vi "ULx Write (Analog 1D DBL 1Chan NSamp).vi"(0 "task in":refnum<k24>, 1 "auto start":bool, 7 "data":dbl[](array[numeric]) format="%0.2f", 9 "timeout":dbl=10.0 format="%_4g", 11 "error in":errorcluster) -> (4 "task out":refnum<k24>, 10 "number of samples written per channel":u32, 15 "error out":errorcluster)   [LabVIEW 2020]
doc: "Writes one or more floating-point samples to a task that contains a single analog output channel."
uses:
  C:/Users/William/Documents/LV 2020 builds/LeaktestDAQ/Source-v33/ULx_LV.dll
  ULx_LV.dll
panel:
  # "sample #"
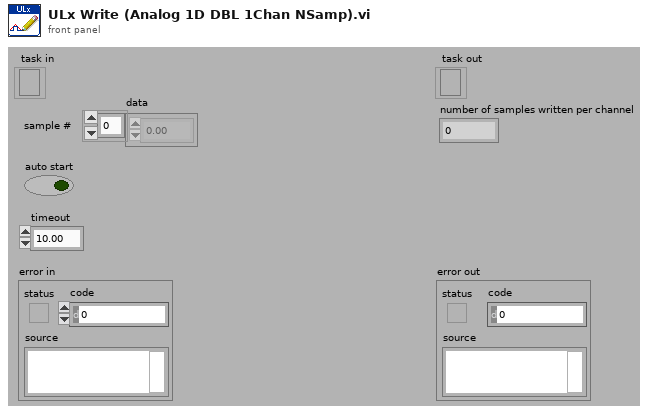
[diagram p1: front panel]
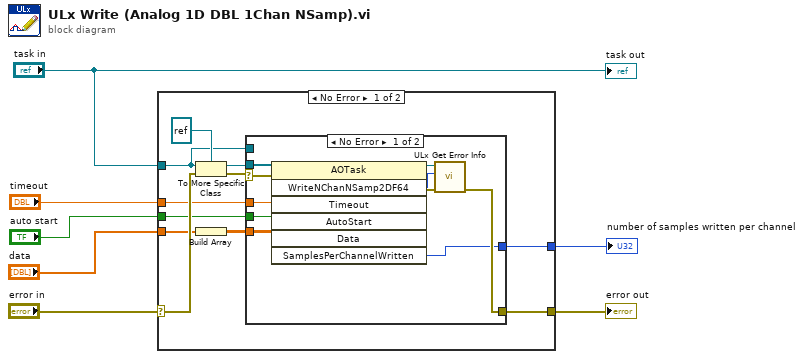
[diagram p0: block diagram]
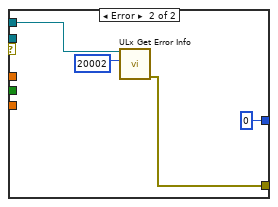
[diagram p2: hidden frame]
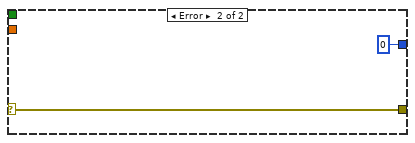
[diagram p3: hidden frame]
diagram:
  n1 = case shown="No Error" "error in" {
    selector: "error in" -> [w18 w34]
    tunnel: "task in" -> [w12 _]
    tunnel: "timeout" -> [w14 _]
    tunnel: [w13 w34] -> w5
    tunnel: "data" -> [w8 _]
    tunnel: "auto start" -> [w11 _]
    tunnel: [w10 0 ("SamplesPerChannelWritten")] -> w1
    frame No Error {
      n2 = To More Specific Class(target class=refnum<k24> refnum, reference=w12, error in=w18) -> (specific class reference=w15:refnum<k24>, error out=w16:errorcluster)
      n3 = Build Array(w8) -> (w9:dbl[][])
      n4 = case shown="No Error" w16 {
        selector: w16 -> [w27 _]
        tunnel: w15 -> [w28 _]
        tunnel: w14 -> [w21 _]
        tunnel: [w24 w31] -> w13
        tunnel: w12 -> [_ w30]
        tunnel: w9 -> [w19 _]
        tunnel: w11 -> [w20 _]
        tunnel: [w22 0 ("SamplesPerChannelWritten")] -> w10
        frame No Error {
          n5 = invoke class="AOTask" method="WriteNChanNSamp2DF64"(reference=w28, error in=w27, "Timeout"=w21, "AutoStart"=w20, "Data"=w19) -> (reference out=w25:refnum<k24>, error out=w26:errorcluster, "WriteNChanNSamp2DF64"=w23:i32, "SamplesPerChannelWritten"=w22:u32)  [unwired: 2 in, 3 out]
          n6 = call "ULx Get Error Info.vi"("error in"=w26, "ErrorCode"=w23, "task in"=w25) -> ("error out"=w24:errorcluster)  [unwired: 8 in]
        }
        frame Error {
          n7 = call "ULx Get Error Info.vi"("ErrorCode"=20002, "task in"=w30) -> ("error out"=w31:errorcluster)  [unwired: 9 in]
        }
      }
    }
    frame Error {
    }
  }
  "error out" <- w5
  "number of samples written per channel" <- w1
  "task out" <- "task in"
